vi "Open Connection to Shared Variables.vi"(8 "Error In":errorcluster, 11 "Page Configurations In":T2(array[cluster])) -> (0 "Error Out":errorcluster, 3 "Page Configurations Out":T2(array[cluster]))   [LabVIEW 2017, in "DTacq Plot Display Library.lvlib"]
doc: "Opens a read-only connection to every shared variable which is a part of this configuration.\n\nA connection to a shared variable must be open, before attempting to read data from it."
uses:
  DTacq Plot Display Library.lvlib
  Typedefs/Plot Channel Configruation--Cluster.ctl
  Network Shared Variables/Typedefs/X and Y Variant Arrays--Cluster.ctl
  Network Shared Variables/Shared Variables Library.lvlib
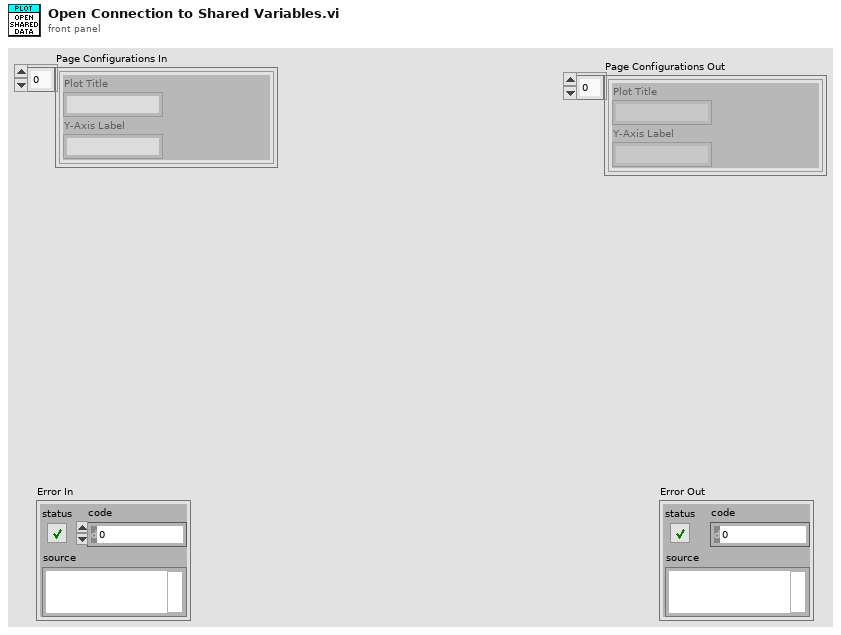
[diagram p1: front panel]
types:
  T1 = typedef "DTacq Plot Display Library.lvlib/Plot Channel Configruation--Cluster.ctl" = cluster{"Shared Variable Reference":refnum<k21>, "Full Variable Name":string, "URL":string, "Descriptive Name":string, "Data Type":variant, "Colour":u32}
  T2 = cluster{"Plot Title":string, "Y-Axis Label":string, "X-Axis Label":string, "Plot Channel Configurations":T1[]}[]
  T3 = typedef "Shared Variables Library.lvlib/X and Y Variant Arrays--Cluster.ctl" = cluster{"X-Data":variant[], "Y-Data":variant[]}
  T4 = cluster{"Read Access":enum8{"Allowed", "Required", "None"}, "Write Access":enum8{"Allowed", "Required", "None"}}
  T5 = cluster{"Plot Title":string, "Y-Axis Label":string, "X-Axis Label":string, "Plot Channel Configurations":T1[]}
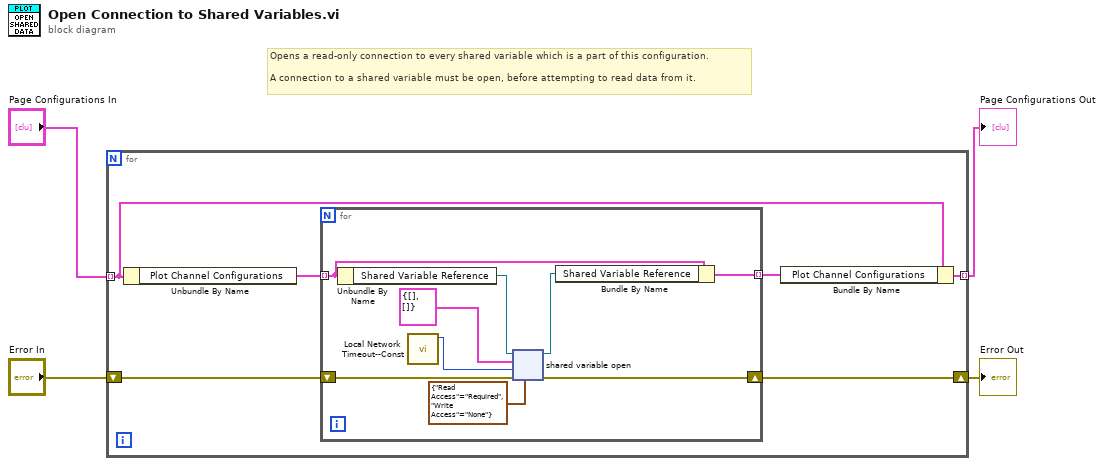
[diagram p0: block diagram]
diagram:
  # "Opens a read-only connection to every shared variable which is a part of this configuration.\n\nA connection to a shared variable must be open, before attempting to read data from it."
  n1 = for {
    tunnel: "Page Configurations In" -> [w7] mode=indexing
    shift-right: [w8] -> w3
    shift-left: "Error In" -> [w9]
    tunnel: [w5] -> w1 mode=indexing
    n2 = Unbundle By Name(w7) -> ("Plot Channel Configurations"=w10:T1[])
    n3 = for {
      tunnel: w10 -> [w18] mode=indexing
      shift-right: [w14] -> w8
      shift-left: w9 -> [w15]
      tunnel: [w13] -> w6 mode=indexing
      n4 = Unbundle By Name(w18) -> ("Shared Variable Reference"=w19:refnum<k21>)
      n5 = call "Local Network Timeout--Const.vi"() -> ("Local Network Timeout (ms)"=w16:i32)  [unwired: 11 in]
      n6 = shared-variable-open(w19, w15, T3 {"X-Data"=[], "Y-Data"=[]} ("Data Cluster"), T4 {"Read Access"=enum."Required", "Write Access"=enum."None"} ("access"), w16) -> (w17:refnum<k21>, w14:errorcluster)  [unwired: 1 in]
      n7 = Bundle By Name(cluster=w18, "Shared Variable Reference"=w17) -> (w13:T1)
    }
    n8 = Bundle By Name(cluster=w7, "Plot Channel Configurations"=w6) -> (w5:T5)
  }
  "Page Configurations Out" <- w1
  "Error Out" <- w3
